vi "SingleCore.vi"(0 "alpha":sgl, 1 "Parameters":T1={"Deadtime"="Deadtime", "Period"="Period"}, 2 "ref_max":sgl=0.9999695, 5 "beta":sgl, 9 "input valid":bool=TRUE, 12 "enable":bool=TRUE) -> (4 "SwitchPositions":T2, 14 "Sector":u8, 15 "ready for input":bool)   [LabVIEW 2017, in "SVPWM.lvlib"]
uses:
  SVPWM.lvlib
  SwitchPositions.ctl
  Parameters.ctl
  <vilib>/Utility/error.llb/Clear Errors.vi
  <vilib>/rvi/Emulation/niFpgaSctlEmulationGetInTimedLoop.vi
  <vilib>/rvi/DataTransferAndStorage/Container/Common/niFpgaContainerExecOnDevCompGetState.vi
  <vilib>/rvi/Emulation/niFpgaEmulationIsFPGAContextNoSignature.vi
  <vilib>/rvi/DataTransferAndStorage/Container/Common/niFpgaContainerGetUniqueNameForEmu.vi
  <vilib>/rvi/Memory/Memory_Emulation/niFpgaMemoryEmulationCacheClearOnFirstRun.vi
  <vilib>/rvi/Memory/Memory_Emulation/nirvimemoryEmulationManagerCache_MakeExclusive.vi
  <vilib>/rvi/Memory/Memory_Emulation/niFpgaMemoryEmulationValidateCache.vi
  <vilib>/rvi/Memory/Memory_Emulation/nirvimemoryEmulationManagerCache_InsertValue.vi
  <vilib>/rvi/Memory/Memory_Emulation/nirvimemoryEmulationManagerCache_ReleaseExclusive.vi
  <vilib>/rvi/Memory/Memory_Emulation/nirvimemoryEmulationManagerCache_GetValue.vi
  <vilib>/rvi/Memory/Memory_Emulation/nirvimemoryEmulationManagerCache_SetValue.vi
  <vilib>/rvi/Emulation/niFpgaProcessEmulError.vi
  <vilib>/rvi/DataTransferAndStorage/Container/XNode/niFpgaContainer.xnode
  <vilib>/rvi/DataTransferAndStorage/Register/Emulation/niFpgaRegisterEmulationRefIn.vi
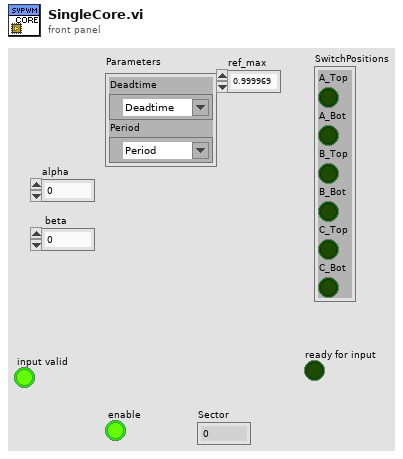
[diagram p1: front panel]
types:
  T1 = typedef "SVPWM.lvlib/Parameters.ctl" = cluster{"Deadtime":refnum<k21>, "Period":refnum<k21>}
  T2 = typedef "SVPWM.lvlib/SwitchPositions.ctl" = cluster{"A_Top":bool, "A_Bot":bool, "B_Top":bool, "B_Bot":bool, "C_Top":bool, "C_Bot":bool}
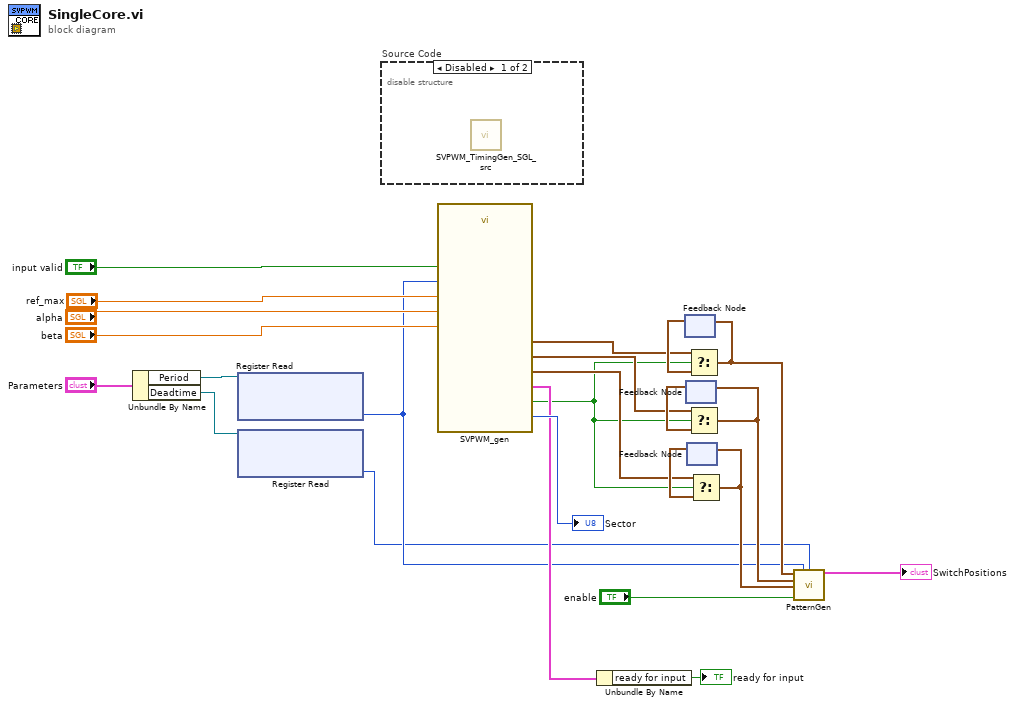
[diagram p0: block diagram]
diagram:
  n1 = Unbundle By Name("Parameters") -> ("Period"=w4:refnum<k21>, "Deadtime"=w3:refnum<k21>)
  n2 = xnode ("Register Read")("Register In"=w4) -> ("Data"=w2:u32)  [unwired: 1 out]
  n3 = xnode ("Register Read")("Register In"=w3) -> ("Data"=w1:u8)  [unwired: 1 out]
  n4 = disable-structure "Source Code" shown="Disabled" {
    frame Disabled {
      n5 = call "SVPWM_TimingGen_SGL_src.vi"() -> ()  [unwired: 12 in, 4 out]
    }
    frame Enabled {
    }
  }
  n6 = call "SVPWM_gen.vi"("ref_beta"="beta", "Period"=w2, "ref_max"="ref_max", "input valid"="input valid", "ref_alpha"="alpha") -> ("Sector"=→"Sector":u8, "C_Timing"=w7:cluster{"ON":u32, "OFF":u32}, "B_timing"=w8:cluster{"ON":u32, "OFF":u32}, "output valid"=w6:bool, "feedback signals"=w10:cluster{"ready for input":bool}, "A_timing"=w9:cluster{"ON":u32, "OFF":u32})  [unwired: 5 in]
  n7 = Unbundle By Name(w10) -> ("ready for input"=→"ready for input":bool)
  n8 = feedback #1() -> (w24:cluster{"ON":u32, "OFF":u32})  [unwired: 1 in]
  n9 = feedback #2() -> (w23:cluster{"ON":u32, "OFF":u32})  [unwired: 1 in]
  n10 = feedback #3() -> (w22:cluster{"ON":u32, "OFF":u32})  [unwired: 1 in]
  n11 = Select(t=w9, s=w6, f=w24) -> (s? t:f=w21:cluster{"ON":u32, "OFF":u32})
  n12 = feedback-in #1(w21) -> ()
  n13 = Select(t=w8, s=w6, f=w23) -> (s? t:f=w20:cluster{"ON":u32, "OFF":u32})
  n14 = feedback-in #2(w20) -> ()
  n15 = Select(t=w7, s=w6, f=w22) -> (s? t:f=w19:cluster{"ON":u32, "OFF":u32})
  n16 = feedback-in #3(w19) -> ()
  n17 = call "PatternGen.vi"("A_timing"=w21, "Period"=w2, "Deadtime"=w1, "B_timing"=w20, "C_timing"=w19, "enable"="enable") -> ("SwitchPositions"=→"SwitchPositions":T2)  [unwired: 9 in]
